vi "Fridge_Valve_Status.vi"() -> (1 "n_ng":u8, 2 "values":T1)   [LabVIEW 2019]
uses:
  Fridge_Valve_Global.vi
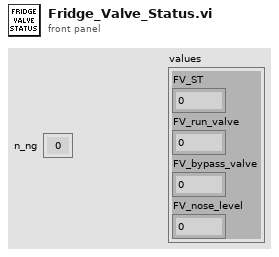
[diagram p1: front panel]
types:
  T1 = cluster{"FV_ST":u32, "FV_run_valve":dbl, "FV_bypass_valve":dbl, "FV_nose_level":dbl}
  T2 = enum32{"Bad", "Idle", "Run top level", "Running"}
  T3 = cluster{"MKS670_1000_ST":u32, "FV_run_valve":dbl, "FV_bypass_valve":dbl, "FV_nose_level":dbl}
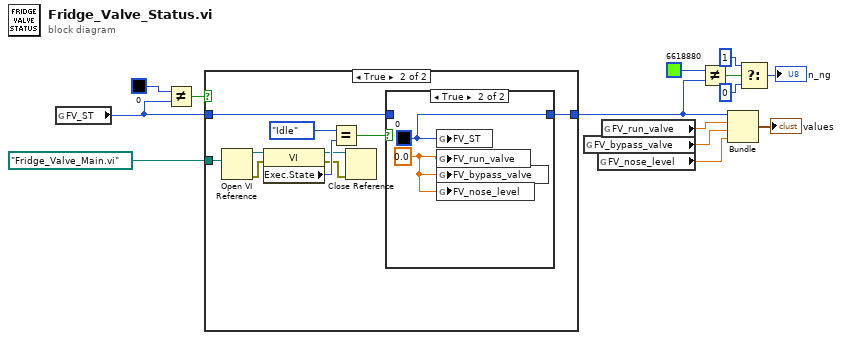
[diagram p0: block diagram]
diagram:
  n1 = global read "Fridge_Valve_Global.vi" "FV_ST"() -> (w5:u32)
  n2 = Not Equal?(x=u32 0 ("MKS670_1000_ST 2"), y=w5) -> (x != y?=w14:bool)
  n3 = case shown="True" w14 {
    tunnel: w5 -> [w15 w17]
    tunnel: [w15 w16] -> w11
    tunnel: path "Fridge_Valve_Main.vi" ("vi path") -> [_ w18]
    frame False {
    }
    frame True {
      n4 = Open VI Reference(vi path=w18) -> (vi reference=w25:refnum<vi>, error out=w24:errorcluster)  [unwired: 5 in]
      n5 = property class="VI"(reference=w25, error in=w24) -> (reference out=w20:refnum<vi>, error out=w19:errorcluster, "Exec.State"=w22:T2)
      n6 = Equal?(x=T2."Idle" ("Execution:State"), y=w22) -> (x = y?=w23:bool)
      n7 = Close Reference(reference=w20, error in (no error)=w19) -> ()  [unwired: 1 out]
      n8 = case shown="True" w23 {
        tunnel: w17 -> [w26 _]
        tunnel: [w26 w28] -> w16
        frame False {
        }
        frame True {
          w27 = 0.0 ("MKS670_1000_P")
          w28 = u32 0 ("MKS670_1000_ST")
          n9 = global write "Fridge_Valve_Global.vi" "FV_ST"(w28) -> ()
          n10 = global write "Fridge_Valve_Global.vi" "FV_run_valve"(w27) -> ()
          n11 = global write "Fridge_Valve_Global.vi" "FV_bypass_valve"(w27) -> ()
          n12 = global write "Fridge_Valve_Global.vi" "FV_nose_level"(w27) -> ()
        }
      }
    }
  }
  n13 = global read "Fridge_Valve_Global.vi" "FV_bypass_valve"() -> (w3:dbl)
  n14 = global read "Fridge_Valve_Global.vi" "FV_nose_level"() -> (w2:dbl)
  n15 = global read "Fridge_Valve_Global.vi" "FV_run_valve"() -> (w4:dbl)
  n16 = Not Equal?(x=u32 6618880 ("MKS670_1000_ST 2"), y=w11) -> (x != y?=w9:bool)
  n17 = Bundle("MKS670_1000_ST"=w11, "FV_run_valve"=w4, "FV_bypass_valve"=w3, "FV_nose_level"=w2) -> (→"values":T3)  [unwired: 1 in]
  n18 = Select(t=u8 1 ("n_ng"), s=w9, f=u8 0 ("n_ng")) -> (s? t:f=→"n_ng":u8)
